vi "extract region of Interest.vi"() -> ()   [LabVIEW 2013]
uses:
  <vilib>/vision/NI_Vision_Development_Module.lvlib
panel:
  out "ROI":T1(plugin-control)
  out "Image":T1(plugin-control)
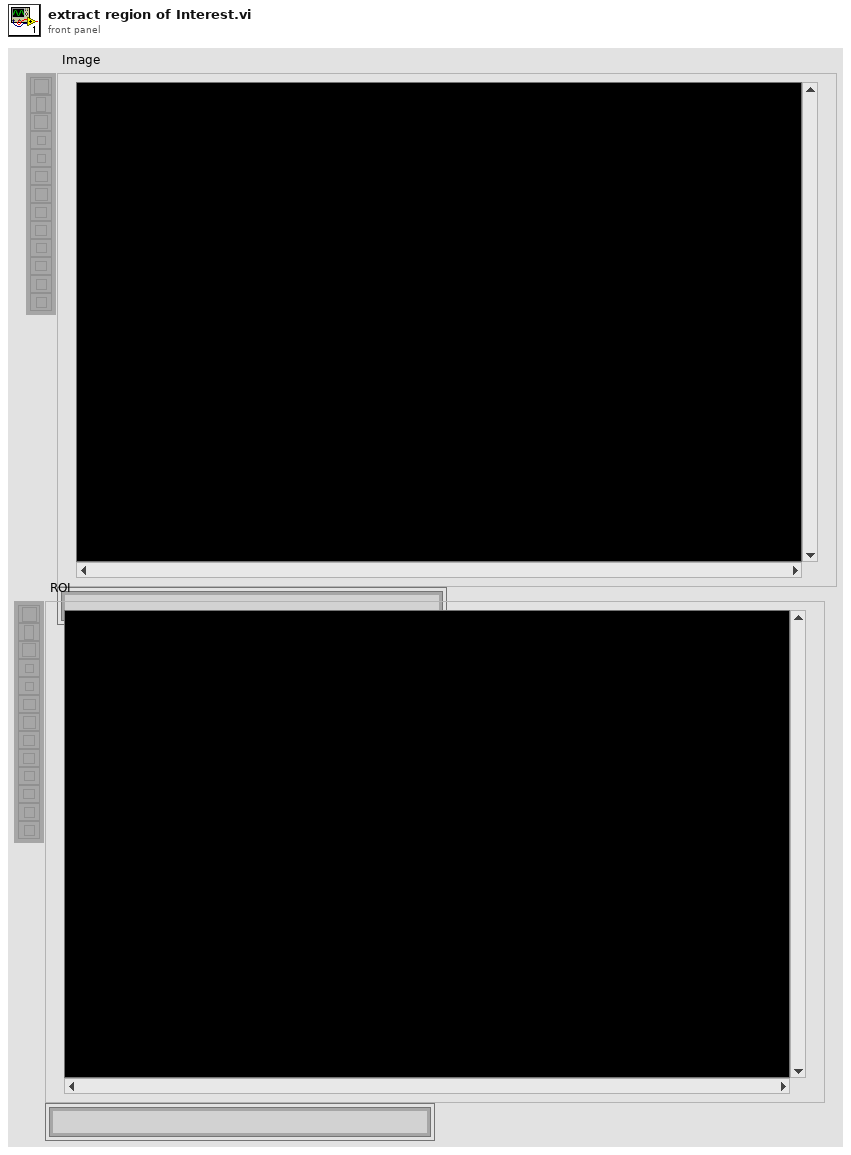
[diagram p1: front panel]
types:
  T1 = typedef "IMAQ Image.ctl" = refnum<image>
  T2 = typedef "Image Type" = u32
  T3 = typedef "IMAQ Rectangle" = cluster{"Left":i32, "Top":i32, "Right":i32, "Bottom":i32, "Rotation":dbl}
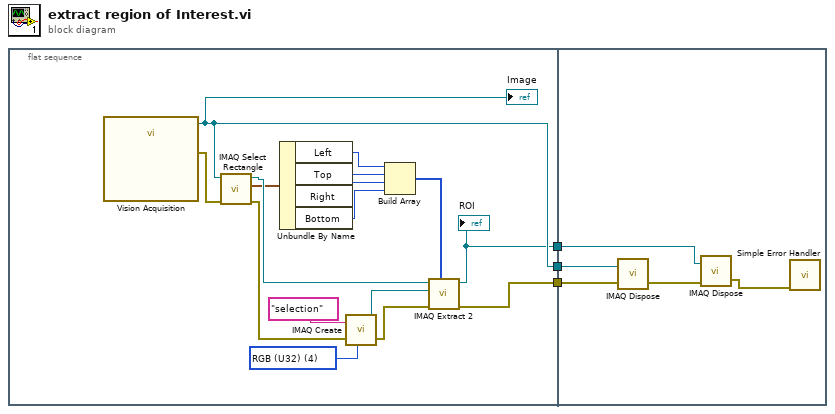
[diagram p0: block diagram]
diagram:
  n1 = flat-sequence {
    tunnel: [w13] -> w3
    tunnel: [w6] -> w2
    tunnel: [w5] -> w1
    tunnel: w3 -> [w23]
    tunnel: w2 -> [w24]
    tunnel: w1 -> [w20]
    frame #0 {
      w4 = T2 4 items=["Grayscale (U8)", "Grayscale (I16)", "Grayscale (SGL)", "Complex (CSG)", "RGB (U32)", "HSL (U32)", "RGB (U64)", "Grayscale (U16)"] ("Image Type")
      n2 = call "Vision Acquisition"() -> ("Image Out"=w6:T1, "error out"=w19:errorcluster)  [unwired: 26 in]
      "Image" <- w6
      n3 = call "IMAQ Select Rectangle"("error in (no error)"=w19, "Image In"=w6) -> ("error out"=w18:errorcluster, "Rectangle"=w12:T3, "Image Out (duplicate)"=w14:T1)  [unwired: 6 in, 1 out]
      n4 = Unbundle By Name(w12) -> ("Left"=w11:i32, "Top"=w10:i32, "Right"=w9:i32, "Bottom"=w8:i32)
      n5 = call "IMAQ Create"("Image Name"="selection", "Image Type"=w4, "error in (no error)"=w18) -> ("New Image"=w15:T1, "error out"=w16:errorcluster)  [unwired: 2 in]
      n6 = Build Array(w11, w10, w9, w8) -> (w7:i32[])
      n7 = call "IMAQ Extract 2"("Optional Rectangle"=w7, "error in (no error)"=w16, "Image Dst"=w15, "Image Src"=w14) -> ("error out"=w13:errorcluster, "Image Dst Out"=w5:T1)  [unwired: 6 in]
      "ROI" <- w5
    }
    frame #1 {
      n8 = call "IMAQ Dispose"("Image"=w24, "error in (no error)"=w23) -> ("error out"=w22:errorcluster)  [unwired: 4 in]
      n9 = call "IMAQ Dispose"("Image"=w20, "error in (no error)"=w22) -> ("error out"=w21:errorcluster)  [unwired: 4 in]
      n10 = call <vilib>:"Simple Error Handler.vi"("error in (no error)"=w21) -> ()  [unwired: 4 in, 5 out]
    }
  }
